vi "CMW_control.vi"() -> ()   [LabVIEW 2013]
uses:
  <vilib>/Utility/file.llb/Write To Spreadsheet File (DBL).vi
panel:
  out "Current Power":dbl
  in  "TT on/off":bool
  out "Reliability Indicator":dbl
  in  "stop":bool
  out "TT":i32
  in  "Start Measurement":bool
  out "RS EPRE":dbl=-40.81
  in  "Idle Cell Power":dbl=-16.0
  out "Measurement time":u32=121989224
  out "Avg TPUT":cluster{dbl[], dbl[]}(graph)={[-9.809999999999999], [0.0]}
  out "Lost Connection":bool
  in  "Stop Power":dbl=-25.0
  in  "Step Power":dbl=1.0
  in  "Start Power":dbl=-15.0
  out "Current Angle":i32=-1
  out "Output Power":string="-1.603879E+001\n"
  out "TPUT":dbl
  out "Connected":bool
  out "Current Throughput":dbl(graph)
  in  "Serial Port":refnum<visa-resource-name>="ASRL4::INSTR"
  out "DCD":bool
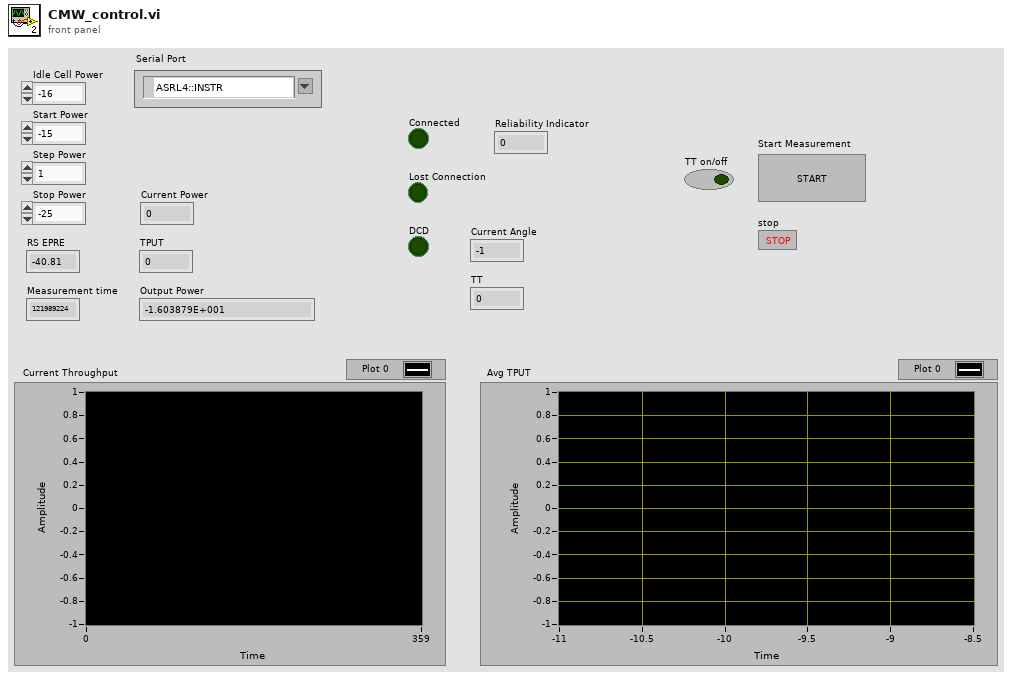
[diagram p1: front panel]
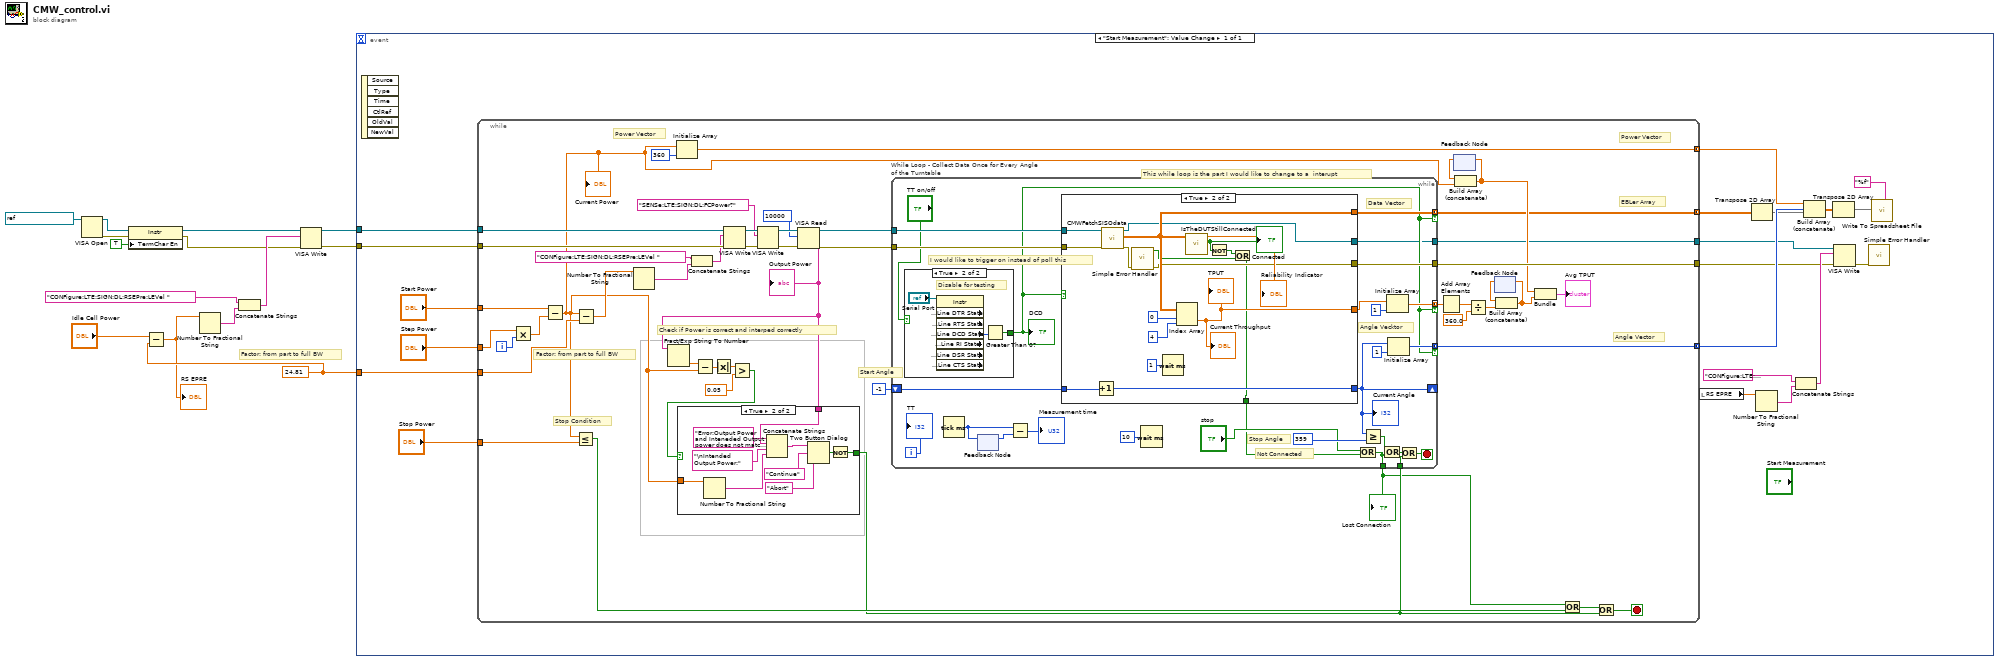
[diagram p0: block diagram]
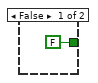
[diagram p2: hidden frame]
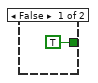
[diagram p3: hidden frame]
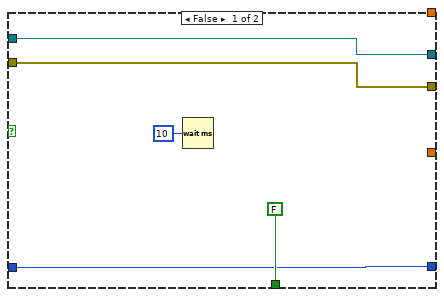
[diagram p4: hidden frame]
diagram:
  w2 = 24.81 ("y")
  # "Factor: from part to full BW"
  n1 = VISA Open(VISA resource name=refnum<visa-resource-name> "CMW500-VXI") -> (VISA resource name=w12:refnum<visa-resource-name>, error out=w11:errorcluster)  [unwired: 4 in]
  n2 = property class="Instr"(reference=w12, error in=w11, "TermChar En"=TRUE ("Message Based Settings:Termination Character Enable")) -> (reference out=w5:refnum<visa-resource-name>, error out=w4:errorcluster)
  n3 = Subtract(x="Idle Cell Power", y=w2) -> (x-y=w1:dbl)
  "RS EPRE" <- w1
  n4 = Number To Fractional String(number=w1) -> (F-format string=w10:string)  [unwired: 3 in]
  n5 = Concatenate Strings("CONFigure:LTE:SIGN:DL:RSEPre:LEVel " ("write buffer"), w10) -> (w9:string)
  n6 = VISA Write(VISA resource name=w5, write buffer=w9, error in (no error)=w4) -> (VISA resource name out=w7:refnum<visa-resource-name>, error out=w6:errorcluster)  [unwired: 1 out]
  n7 = event shown="[0] \"Start Measurement\": Value Change" {
    selector: _ -> [_]
    dyn-events: _ -> [_]
    timeout: _ -> [_]
    tunnel: w7 -> [w34]
    tunnel: w6 -> [w33]
    tunnel: w2 -> [w22]
    event "Start Measurement": Value Change {
      n8 = event-data() -> ()  [unwired: 1 in, 6 out]
      n9 = while {
        tunnel: w34 -> [w82]
        tunnel: w33 -> [w81]
        tunnel: [w72] -> w15
        tunnel: "Start Power" -> [w66]
        tunnel: "Step Power" -> [w64]
        tunnel: "Stop Power" -> [w54]
        tunnel: [w48] -> w28 mode=concatenating
        tunnel: [w42] -> w29 mode=concatenating
        tunnel: [w41] -> w27 mode=concatenating
        tunnel: w22 -> [w37]
        tunnel: [w36] -> w18
        i -> [w65]
        stop <- w55 stop-if-true
        # "This while loop is the part I would like to change to a  interupt"
        # "Start Angle"
        # "Angle Vector"
        # "EBLer Array"
        # "Power Vector"
        # "Power Vector"
        # "Stop Condition"
        # "Check if Power is correct and interped correctly"
        # "Factor: from part to full BW"
        n10 = Multiply(x=w64, y=w65) -> (x*y=w63:dbl)
        n11 = Subtract(x=w66, y=w63) -> (x-y=w35:dbl)
        "Current Power" <- w35
        n12 = Less Or Equal?(x=w35, y=w54) -> (x <= y?=w53:bool)
        n13 = Subtract(x=w35, y=w37) -> (x-y=w46:dbl)
        n14 = Number To Fractional String(number=w46) -> (F-format string=w58:string)  [unwired: 3 in]
        n15 = Initialize Array(w35, 360 ("dimension size")) -> (w48:dbl[])
        n16 = Concatenate Strings("CONFigure:LTE:SIGN:DL:RSEPre:LEVel " ("write buffer"), w58) -> (w70:string)
        n17 = VISA Write(VISA resource name=w82, write buffer=w70, error in (no error)=w81) -> (VISA resource name out=w80:refnum<visa-resource-name>, error out=w78:errorcluster)  [unwired: 1 out]
        n18 = VISA Write(VISA resource name=w80, write buffer="SENSe:LTE:SIGN:DL:FCPower?", error in (no error)=w78) -> (VISA resource name out=w77:refnum<visa-resource-name>, error out=w76:errorcluster)  [unwired: 1 out]
        n19 = VISA Read(VISA resource name=w77, byte count=u32 10000, error in (no error)=w76) -> (VISA resource name out=w74:refnum<visa-resource-name>, read buffer=w60:string, error out=w73:errorcluster)  [unwired: 1 out]
        "Output Power" <- w60
        n20 = Fract/Exp String To Number(string=w60) -> (number=w59:dbl)  [unwired: 3 in, 1 out]
        n21 = Subtract(x=w59, y=w35) -> (x-y=w62:dbl)
        n22 = Absolute Value(x=w62) -> (abs(x)=w61:dbl)
        n23 = Greater?(x=w61, y=0.05) -> (0:w56:bool)
        n24 = case shown="True" w56 {
          tunnel: w60 -> [_ w92]
          tunnel: w35 -> [_ w86]
          tunnel: [FALSE w84] -> w39
          frame False {
          }
          frame True {
            n25 = Number To Fractional String(number=w86) -> (F-format string=w90:string)  [unwired: 3 in]
            n26 = Concatenate Strings("Error:Output Power and Inteneded Output power does not match:\nOutput Power:" ("write buffer"), w92, "\nIntended Output Power:" ("write buffer"), w90) -> (w89:string)
            n27 = Two Button Dialog(message=w89, 1:"Abort" ("F button name (\"Cancel\")"), 2:"Continue" ("T button name (\"OK\")")) -> (T button?=w85:bool)
            n28 = Not(x=w85) -> (.not. x?=w84:bool)
          }
        }
        n29 = while "While Loop - Collect Data Once for Every Angle of the Turntable" {
          tunnel: w74 -> [w120]
          tunnel: w73 -> [w119]
          tunnel: [w118] -> w72
          tunnel: [w115] -> w42 mode=concatenating if=w109
          tunnel: [w113] -> w41 mode=concatenating if=w109
          tunnel: [w98] -> w38
          tunnel: [w110] -> w69 mode=concatenating if=w109
          shift-right: [w108] -> _
          shift-left: -1 ("index") -> [w107]
          tunnel: w39 -> [w105]
          tunnel: [w101] -> w36
          i -> [w100]
          stop <- w99 stop-if-true
          # "I would like to trigger on instead of poll this"
          # "Data Vector"
          # "Angle Vecktor"
          # "Not Connected"
          # "Stop Angle"
          n30 = case shown="True" "TT on/off" {
            tunnel: [TRUE w124] -> w109
            frame False {
            }
            frame True {
              # "Disable for testing"
              n31 = property class="Instr" props=["Serial Settings:Modem Line Settings:Line DTR State", "Serial Settings:Modem Line Settings:Line RTS State", "Serial Settings:Modem Line Settings:Line DCD State", "Serial Settings:Modem Line Settings:Line RI State", "Serial Settings:Modem Line Settings:Line DSR State", "Serial Settings:Modem Line Settings:Line CTS State"](reference="Serial Port") -> ("Serial Settings:Modem Line Settings:Line DCD State"=w123:i16)  [unwired: 1 in, 7 out]
              n32 = Greater Than 0?(x=w123) -> (x > 0?=w124:bool)
            }
          }
          "DCD" <- w109
          n33 = Tick Count (ms)() -> (millisecond timer value=w103:u32)
          n34 = feedback-in #1(w103) -> ()
          n35 = feedback #1() -> (w102:u32)  [unwired: 1 in]
          n36 = Subtract(x=w103, y=w102) -> (x-y=→"Measurement time":u32)
          n37 = case shown="True" w109 {
            tunnel: w120 -> [w126 w144]
            tunnel: w119 -> [w129 w143]
            tunnel: [w129 w135] -> w118
            tunnel: [_ w142] -> w115
            tunnel: [w127 w141] -> w108
            tunnel: [FALSE ("Connected") w130] -> w94
            tunnel: [_ w140] -> w111
            tunnel: w107 -> [w127 w139]
            tunnel: [w126 w138] -> w101
            frame False {
              n38 = Wait (ms)(milliseconds to wait=u32 10) -> ()  [unwired: 1 out]
            }
            frame True {
              n39 = Increment(x=w139) -> (x+1=w141:i32)
              n40 = call "CMWFetchSISOdata.vi"("error in (no error)"=w143, "VISA Refnum in"=w144) -> ("error out"=w136:errorcluster, "EBLer"=w142:dbl[][], "VISA Refnum out"=w138:refnum<visa-resource-name>)  [unwired: 7 in]
              n41 = call <vilib>:"Simple Error Handler.vi"("error in (no error)"=w136) -> ("error?"=w133:bool, "error out"=w135:errorcluster)  [unwired: 4 in, 3 out]
              n42 = Wait (ms)(milliseconds to wait=u32 1) -> ()  [unwired: 1 out]
              n43 = Index Array(array=w142, index (row)=0 ("index"), index (col)=4 ("disabled index (col)")) -> (element=w140:dbl)
              "Current Throughput" <- w140
              "TPUT" <- w140
              n44 = call "IsTheDUTStillConnected.vi"("EBLer"=w142) -> ("Connected"=w132:bool, "Reliability Indicator"=→"Reliability Indicator":dbl)  [unwired: 9 in]
              "Connected" <- w132
              n45 = Not(x=w132) -> (.not. x?=w131:bool)
              n46 = Or(x=w131, y=w133) -> (x .or. y?=w130:bool)
            }
          }
          "Current Angle" <- w108
          n47 = Wait (ms)(milliseconds to wait=u32 10) -> ()  [unwired: 1 out]
          n48 = Or(x="stop", y=w94) -> (x .or. y?=w98:bool)
          n49 = Greater Or Equal?(x=w108, y=359 ("index")) -> (x >= y?=w117:bool)
          n50 = Or(x=w117, y=w98) -> (x .or. y?=w106:bool)
          n51 = Initialize Array(w111, 1 ("dimension size")) -> (w110:dbl[])
          n52 = Initialize Array(w108, 1 ("dimension size")) -> (w113:i32[])
          n53 = Or(x=w106, y=w105) -> (x .or. y?=w99:bool)
          "TT" <- w100
        }
        "Lost Connection" <- w38
        n54 = Add Array Elements(numeric array=w69) -> (sum=w68:dbl)
        n55 = feedback #2() -> (w47:dbl[])  [unwired: 1 in]
        n56 = Build Array (concatenate)(w47, w35) -> (w44:dbl[])
        n57 = feedback-in #2(w44) -> ()
        n58 = Divide(x=w68, y=360.0) -> (x/y=w49:dbl)
        n59 = feedback #3() -> (w50:dbl[])  [unwired: 1 in]
        n60 = Build Array (concatenate)(w50, w49) -> (w43:dbl[])
        n61 = feedback-in #3(w43) -> ()
        n62 = Bundle(w44, w43) -> (→"Avg TPUT":cluster{dbl[], dbl[]})  [unwired: 1 in]
        n63 = Or(x=w38, y=w53) -> (x .or. y?=w52:bool)
        n64 = Or(x=w52, y=w39) -> (x .or. y?=w55:bool)
      }
      n65 = local read "RS EPRE"() -> (w17:dbl)
      n66 = Transpose 2D Array(2D array=w29) -> (transposed array=w26:dbl[][])
      n67 = Number To Fractional String(number=w17) -> (F-format string=w21:string)  [unwired: 3 in]
      n68 = Concatenate Strings("CONFigure:LTE:SIGN:DL:RSEPre:LEVel " ("write buffer"), w21) -> (w20:string)
      n69 = Build Array (concatenate)(w28, w27, w26) -> (w25:dbl[][])
      n70 = Transpose 2D Array(2D array=w25) -> (transposed array=w24:dbl[][])
      n71 = VISA Write(VISA resource name=w18, write buffer=w20, error in (no error)=w15) -> (error out=w16:errorcluster)  [unwired: 2 out]
      n72 = call <vilib>:"Simple Error Handler.vi"("error in (no error)"=w16) -> ()  [unwired: 4 in, 5 out]
      n73 = call-poly <vilib>:"Write To Spreadsheet File.vi"("format (%.3f)"="%f", "2D data"=w24) -> ()  [unwired: 6 in, 1 out]
    }
  }
